vi "Modelloberfläche.vi"() -> ()   [LabVIEW 2018]
panel:
  out "Fehlermeldung":string
  in  "Variation":string="3,0#3,1#3,2#3,3#3,4#3,6#3,8#4,0#4,1#4,4#4,7"
  out "standard output":string="8.954435503321027e+16 1.6214774937357826e+19 301.81243213234205 38832.501848342836 60.0 78.55471030398478 0.5110838095904991 0.5670084295402535 0.138973917854045\r\n6.941917419433594\r\n" caption="Standardausgabe"
  in  "Simulation starten":bool
  in  "Strom [mA]":dbl=100.0
  out "?":string="RF Leistung [W]"
  in  "Fluss [mg/s]":dbl=8.0
  in  "RF Leistung [W]":dbl=100.0
  in  "Was soll variiert werden?":bool=TRUE
  in  "Abstand Gitter [m]":dbl=0.001
  in  "Gitterspannung [V]":dbl=1000.0
  in  "Widerstand [Ohm]":dbl=2.0
  in  "Windungen":dbl=5.0
  in  "Frequenz [MHz]":dbl=0.5
  in  "Beta g":dbl=0.3
  in  "Beta i":dbl=0.7
  in  "Länge [m]":dbl=0.1
  in  "Radius [m]":dbl=0.06
  in  "Variation oder Performancekurve ?":bool
  in  "Treibstoff":bool
  # "Iod"
  # "Krypton"
  # "Variation"
  # "Performance"
  # "Fluss"
  # "RF Leistung"
  # "Variation von:"
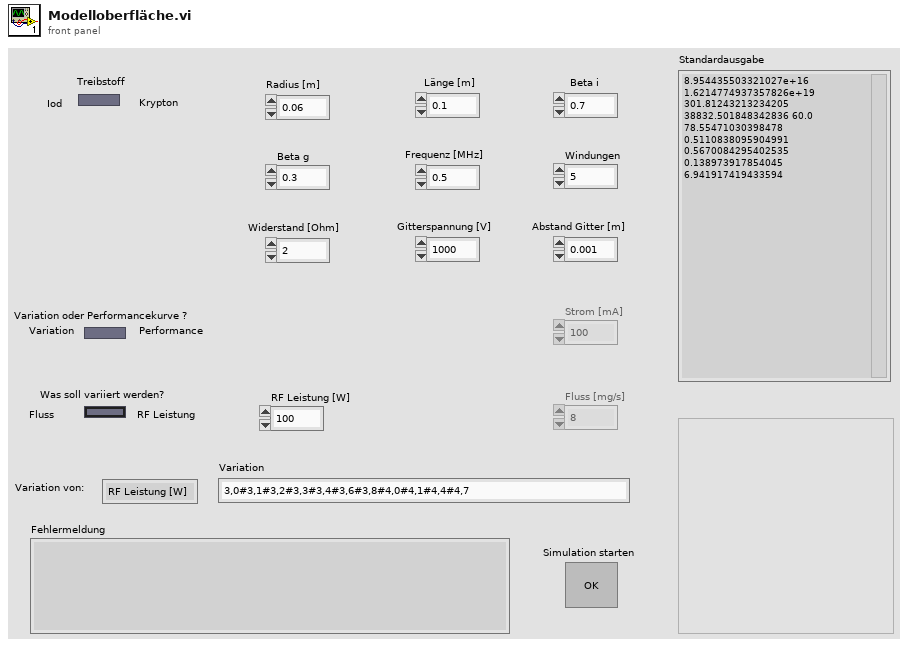
[diagram p1: front panel]
types:
  T1 = enum8{"Enabled", "Disabled", "Disabled and Grayed Out"}
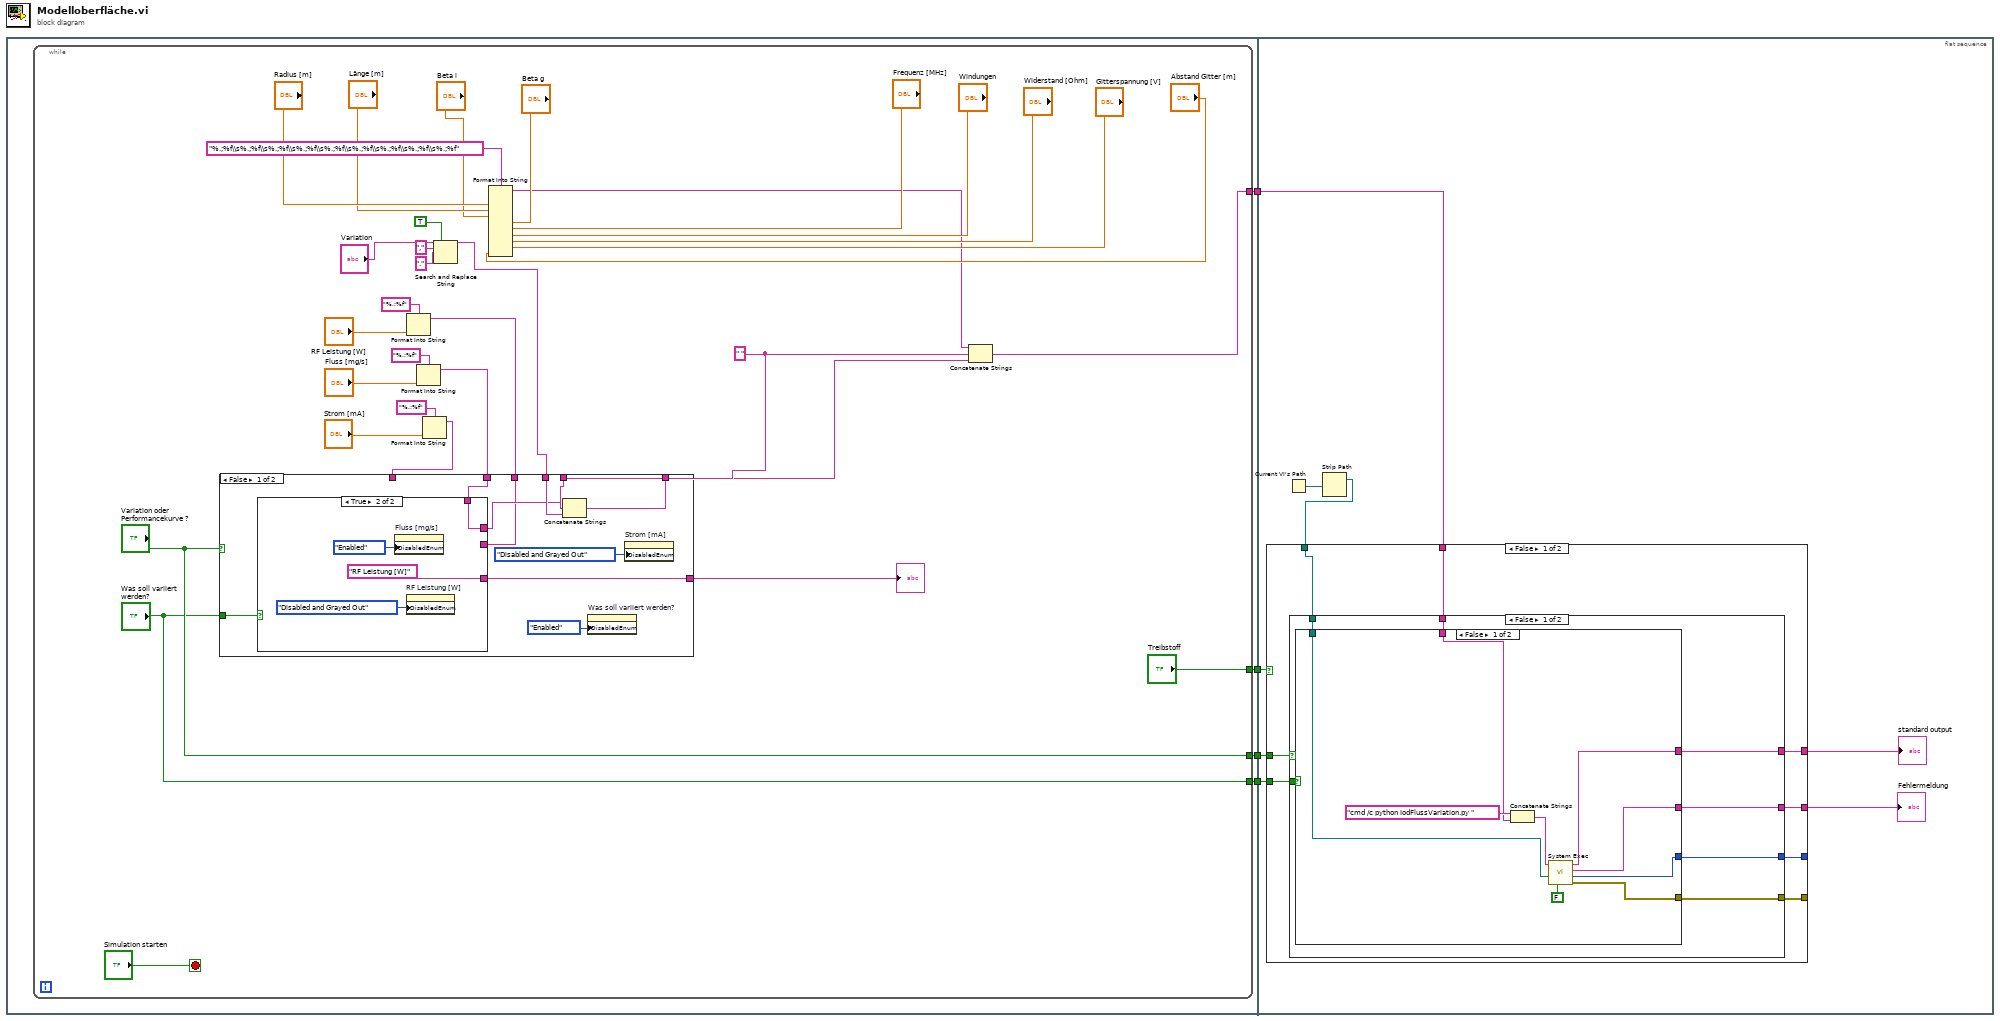
[diagram p0: block diagram]
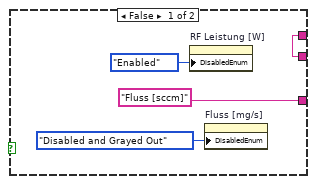
[diagram p2: hidden frame]
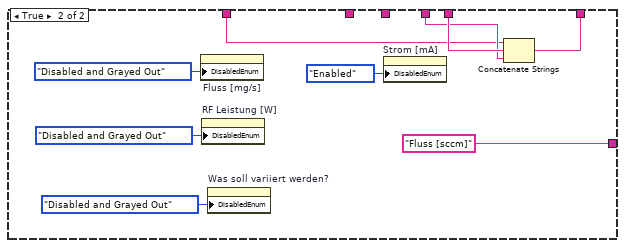
[diagram p3: hidden frame]
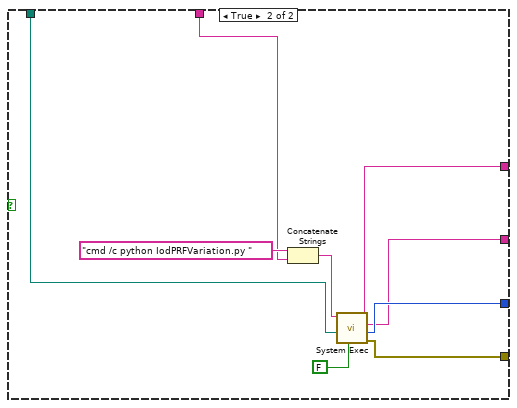
[diagram p4: hidden frame]
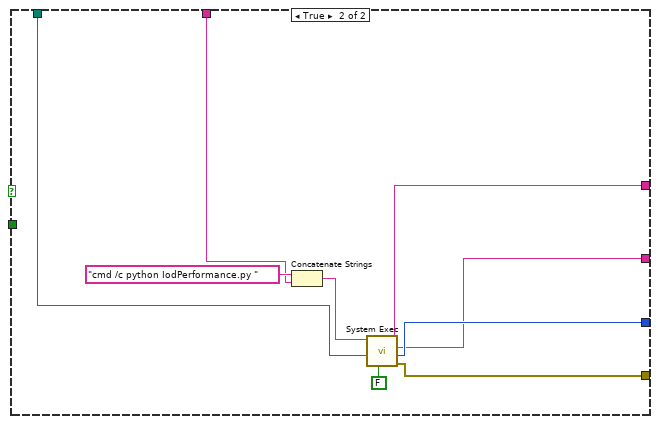
[diagram p5: hidden frame]
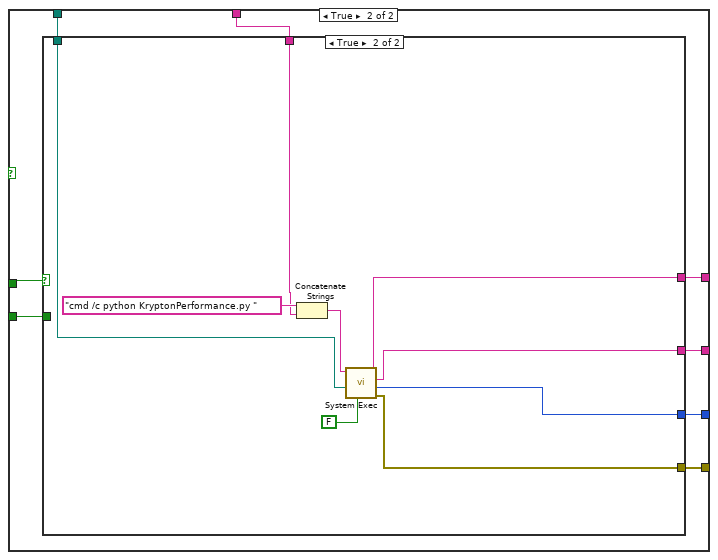
[diagram p6: hidden frame]
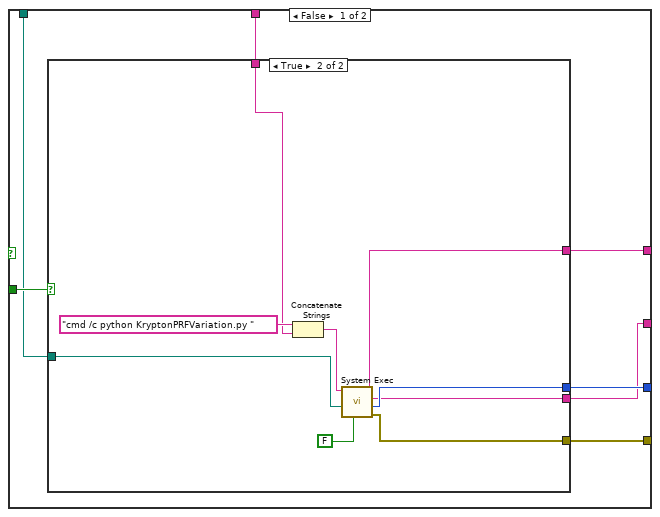
[diagram p7: hidden frame]
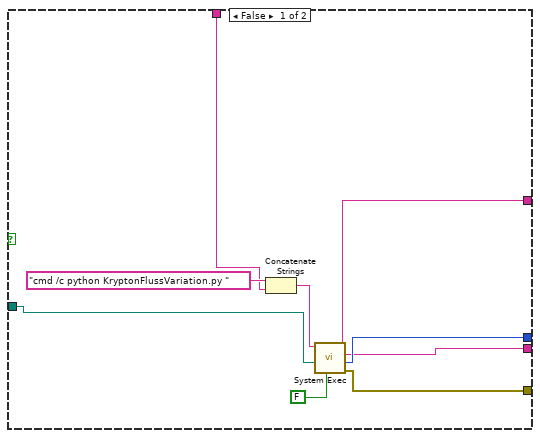
[diagram p8: hidden frame]
diagram:
  n1 = flat-sequence {
    tunnel: [w8] -> w4
    tunnel: [w7] -> w3
    tunnel: [w6] -> w2
    tunnel: [w5] -> w1
    tunnel: w4 -> [w76]
    tunnel: w3 -> [w75]
    tunnel: w2 -> [w74]
    tunnel: w1 -> [w73]
    frame #0 {
      n2 = while {
        tunnel: [w19] -> w8
        tunnel: ["Variation oder Performancekurve ?"] -> w7
        tunnel: ["Was soll variiert werden?"] -> w6
        tunnel: ["Treibstoff"] -> w5
        stop <- "Simulation starten" stop-if-true
        w20 = " "
        n3 = Format Into String(format string="%.;%f" ("Format-String"), "RF Leistung [W]") -> (resulting string=w17:string)  [unwired: 2 in, 1 out]
        n4 = Format Into String(format string="%.;%f" ("Format-String"), "Fluss [mg/s]") -> (resulting string=w22:string)  [unwired: 2 in, 1 out]
        n5 = Format Into String(format string="%.;%f" ("Format-String"), "Strom [mA]") -> (resulting string=w23:string)  [unwired: 2 in, 1 out]
        n6 = Search and Replace String(replace all?=TRUE ("Alle ersetzen? (F)"), input string="Variation", search string="," ("Such-String"), replace string="." ("Ersetzungs-String (\"\")")) -> (result string=w15:string)  [unwired: 4 in, 3 out]
        n7 = case shown="False" "Variation oder Performancekurve ?" {
          tunnel: "Was soll variiert werden?" -> [w51 _]
          tunnel: [w48 "Fluss [sccm]"] -> w30
          tunnel: w15 -> [w45 w62]
          tunnel: [w47 w61] -> w18
          tunnel: w23 -> [_ w60]
          tunnel: w22 -> [w42 _]
          tunnel: w17 -> [w43 _]
          tunnel: w20 -> [w46 w63]
          frame False {
            n8 = case shown="True" w51 {
              tunnel: ["Fluss [sccm]" "RF Leistung [W]"] -> w48
              tunnel: w42 -> [_ w56]
              tunnel: [w52 w56] -> w44
              tunnel: w43 -> [w52 _]
              frame False {
                n9 = property on="RF Leistung [W]" class="DigWert (strikt)"("DisabledEnum"=T1."Enabled" ("Deaktiviert")) -> ()  [unwired: 2 in, 2 out]
                n10 = property on="Fluss [mg/s]" class="DigWert (strikt)"("DisabledEnum"=T1."Disabled and Grayed Out" ("Deaktiviert")) -> ()  [unwired: 2 in, 2 out]
              }
              frame True {
                n11 = property on="Fluss [mg/s]" class="DigWert (strikt)"("DisabledEnum"=T1."Enabled" ("Deaktiviert")) -> ()  [unwired: 2 in, 2 out]
                n12 = property on="RF Leistung [W]" class="DigWert (strikt)"("DisabledEnum"=T1."Disabled and Grayed Out" ("Deaktiviert")) -> ()  [unwired: 2 in, 2 out]
              }
            }
            n13 = Concatenate Strings(w44, w46, w45) -> (w47:string)
            n14 = property on="Was soll variiert werden?" class="Bool. (strikt)"("DisabledEnum"=T1."Enabled" ("Deaktiviert")) -> ()  [unwired: 2 in, 2 out]
            n15 = property on="Strom [mA]" class="DigWert (strikt)"("DisabledEnum"=T1."Disabled and Grayed Out" ("Deaktiviert")) -> ()  [unwired: 2 in, 2 out]
          }
          frame True {
            n16 = property on="Fluss [mg/s]" class="DigWert (strikt)"("DisabledEnum"=T1."Disabled and Grayed Out" ("Deaktiviert")) -> ()  [unwired: 2 in, 2 out]
            n17 = property on="RF Leistung [W]" class="DigWert (strikt)"("DisabledEnum"=T1."Disabled and Grayed Out" ("Deaktiviert")) -> ()  [unwired: 2 in, 2 out]
            n18 = property on="Was soll variiert werden?" class="Bool. (strikt)"("DisabledEnum"=T1."Disabled and Grayed Out" ("Deaktiviert")) -> ()  [unwired: 2 in, 2 out]
            n19 = property on="Strom [mA]" class="DigWert (strikt)"("DisabledEnum"=T1."Enabled" ("Deaktiviert")) -> ()  [unwired: 2 in, 2 out]
            n20 = Concatenate Strings(w60, w63, w62) -> (w61:string)
          }
        }
        "?" <- w30
        n21 = Format Into String(format string="%.;%f\\s%.;%f\\s%.;%f\\s%.;%f\\s%.;%f\\s%.;%f\\s%.;%f\\s%.;%f\\s%.;%f" ("Format-String"), "Radius [m]", "Länge [m]", "Beta i", "Beta g", "Frequenz [MHz]", "Windungen", "Widerstand [Ohm]", "Gitterspannung [V]", "Abstand Gitter [m]") -> (resulting string=w21:string)  [unwired: 2 in, 1 out]
        n22 = Concatenate Strings(w21, w20, w18) -> (w19:string)
      }
    }
    frame #1 {
      n23 = Current VI's Path() -> (path=w70:path)
      n24 = Strip Path(path=w70) -> (stripped path=w69:path)  [unwired: 1 out]
      n25 = case shown="False" w73 {
        tunnel: w76 -> [w84 w126]
        tunnel: w75 -> [w83 w125]
        tunnel: w74 -> [w82 w124]
        tunnel: [w81 w123] -> _
        tunnel: [w80 w122] -> _
        tunnel: [w79 w121] -> w71
        tunnel: [w78 w120] -> w72
        tunnel: w69 -> [w77 w119]
        frame False {
          n26 = case shown="False" w83 {
            tunnel: w84 -> [w91 w115]
            tunnel: w82 -> [w90 _]
            tunnel: [w89 w114] -> w81
            tunnel: [w88 w113] -> w80
            tunnel: [w87 w112] -> w79
            tunnel: [w86 w111] -> w78
            tunnel: w77 -> [w85 w110]
            frame False {
              n27 = case shown="False" w90 {
                tunnel: w91 -> [w97 w106]
                tunnel: [w96 w105] -> w89
                tunnel: [w95 w104] -> w88
                tunnel: [w94 w103] -> w87
                tunnel: [w93 w102] -> w86
                tunnel: w85 -> [w92 w101]
                frame False {
                  n28 = Concatenate Strings("cmd /c python IodFlussVariation.py " ("String"), w97) -> (w100:string)
                  n29 = call <vilib>:"System Exec.vi"("run minimized? (F)"=FALSE, "working directory"=w92, "command line"=w100) -> ("error out"=w96:errorcluster, "return code"=w95:i32, "standard error"=w94:string, "standard output"=w93:string)  [unwired: 5 in]
                }
                frame True {
                  n30 = Concatenate Strings("cmd /c python IodPRFVariation.py " ("String"), w106) -> (w109:string)
                  n31 = call <vilib>:"System Exec.vi"("run minimized? (F)"=FALSE, "working directory"=w101, "command line"=w109) -> ("error out"=w105:errorcluster, "return code"=w104:i32, "standard error"=w103:string, "standard output"=w102:string)  [unwired: 5 in]
                }
              }
            }
            frame True {
              n32 = Concatenate Strings("cmd /c python IodPerformance.py " ("String"), w115) -> (w118:string)
              n33 = call <vilib>:"System Exec.vi"("run minimized? (F)"=FALSE, "working directory"=w110, "command line"=w118) -> ("error out"=w114:errorcluster, "return code"=w113:i32, "standard error"=w112:string, "standard output"=w111:string)  [unwired: 5 in]
            }
          }
        }
        frame True {
          n34 = case shown="True" w125 {
            tunnel: w126 -> [w133 w157]
            tunnel: w124 -> [w132 _]
            tunnel: [w131 w156] -> w123
            tunnel: [w130 w155] -> w122
            tunnel: [w129 w154] -> w121
            tunnel: [w128 w153] -> w120
            tunnel: w119 -> [w127 w152]
            frame False {
              n35 = case shown="True" w132 {
                tunnel: w133 -> [w139 w148]
                tunnel: [w138 w147] -> w131
                tunnel: [w137 w146] -> w130
                tunnel: [w136 w145] -> w129
                tunnel: [w135 w144] -> w128
                tunnel: w127 -> [w134 w143]
                frame False {
                  n36 = Concatenate Strings("cmd /c python KryptonFlussVariation.py " ("String"), w139) -> (w142:string)
                  n37 = call <vilib>:"System Exec.vi"("run minimized? (F)"=FALSE, "working directory"=w134, "command line"=w142) -> ("error out"=w138:errorcluster, "return code"=w137:i32, "standard error"=w136:string, "standard output"=w135:string)  [unwired: 5 in]
                }
                frame True {
                  n38 = Concatenate Strings("cmd /c python KryptonPRFVariation.py " ("String"), w148) -> (w151:string)
                  n39 = call <vilib>:"System Exec.vi"("run minimized? (F)"=FALSE, "working directory"=w143, "command line"=w151) -> ("error out"=w147:errorcluster, "return code"=w146:i32, "standard error"=w145:string, "standard output"=w144:string)  [unwired: 5 in]
                }
              }
            }
            frame True {
              n40 = Concatenate Strings("cmd /c python KryptonPerformance.py " ("String"), w157) -> (w160:string)
              n41 = call <vilib>:"System Exec.vi"("run minimized? (F)"=FALSE, "working directory"=w152, "command line"=w160) -> ("error out"=w156:errorcluster, "return code"=w155:i32, "standard error"=w154:string, "standard output"=w153:string)  [unwired: 5 in]
            }
          }
        }
      }
      "standard output" <- w72
      "Fehlermeldung" <- w71
    }
  }
